vi "GetDataEventProperties.vi"(8 "error in (no error)":errorcluster, 9 "data":T2, 10 "Ir Data Event":T7, 11 "config":T6) -> (0 "error out":errorcluster, 1 "Timestamp":i64, 2 "Props":T1[](array[typedef]), 3 "AssetNodeId":string)   [LabVIEW 2017, in "IrDataEventCreator.lvlib"]
uses:
  <vilib>/addons/InsightCM/Devices/Shared/Ir/IrDataEventCreator/IrDataEventCreator.lvlib
  <vilib>/addons/InsightCM/Devices/Shared/Ir/IrDataEventCreator/controls/IrDataEvent.ctl
  <vilib>/addons/InsightCM/Devices/Shared/Common/DataEvent/controls/EventReference.ctl
  <vilib>/addons/InsightCM/Devices/Shared/Common/DataEvent/controls/Event.ctl
  <vilib>/addons/InsightCM/MessageBus/Base/controls/DataEvent.ctl
  <vilib>/addons/InsightCM/MessageBus/Base/controls/KeyValuePair.ctl
  <vilib>/addons/InsightCM/Devices/Shared/Common/DataEvent/controls/DataSet.ctl
  <vilib>/addons/InsightCM/MessageBus/Base/controls/DataSetMetadata.ctl
  <vilib>/addons/InsightCM/MessageBus/Base/controls/TrendPoint.ctl
  <vilib>/addons/InsightCM/MessageBus/Base/controls/TrendAlarmUpdate.ctl
  <vilib>/addons/InsightCM/MessageBus/Base/controls/TrendAlarmTransition.ctl
  <vilib>/addons/PointValueMap/controls/PointMap.ctl
  <vilib>/addons/InsightCM/Devices/Shared/Ir/IrDataEventCreator/controls/config.ctl
  <vilib>/addons/InsightCM/Devices/Shared/Common/DataFlow/controls/Data.ctl
  <vilib>/addons/InsightCM/Utilities/DataAccessors/controls/wfmSGL_DVR.ctl
  <vilib>/addons/InsightCM/Devices/Shared/Common/DataFlow/controls/Type.ctl
  <vilib>/addons/InsightCM/Utilities/PropertyHelpers/PropertyHelpers.lvlib
  <vilib>/addons/InsightCM/Devices/Shared/Common/DataEvent/DataEvent.lvlib
  <vilib>/addons/PointValueMap/PointValueMap.lvlib
  <vilib>/addons/InsightCM/Devices/Shared/Common/DataFlow/DataFlow.lvlib
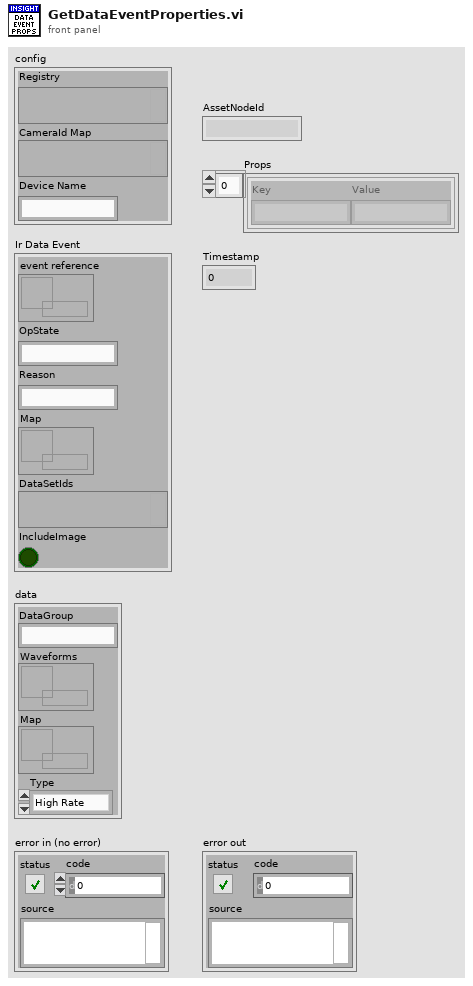
[diagram p1: front panel]
types:
  T1 = typedef "KeyValuePair.ctl" = cluster{"Key":string, "Value":string}
  T2 = typedef "DataFlow.lvlib/Data.ctl" = cluster{"DataGroup":string, "Waveforms":T3, "Map":T4, "Type":T5}
  T3 = typedef "wfmSGL_DVR.ctl" = refnum<data-value>
  T4 = typedef "PointValueMap.lvlib/PointMap.ctl" = refnum<data-value>
  T5 = typedef "DataFlow.lvlib/Type.ctl" = enum16{"High Rate", "Low Rate", "Burst Mode"}
  T6 = typedef "IrDataEventCreator.lvlib/config.ctl" = cluster{"Registry":variant, "CameraId Map":variant, "Device Name":string}
  T7 = typedef "IrDataEventCreator.lvlib/IrDataEvent.ctl" = cluster{"event reference":T8, "OpState":string, "Reason":string, "Map":T4, "DataSetIds":variant, "IncludeImage":bool}
  T8 = typedef "DataEvent.lvlib/EventReference.ctl" = refnum<data-value>
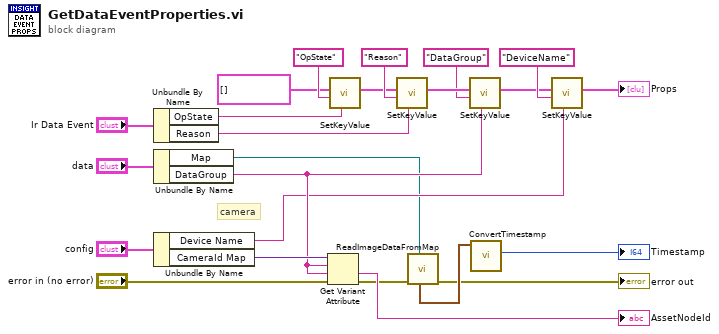
[diagram p0: block diagram]
diagram:
  # "camera"
  n1 = Unbundle By Name("Ir Data Event") -> ("OpState"=w6:string, "Reason"=w16:string)
  n2 = Unbundle By Name("data") -> ("Map"=w4:T4, "DataGroup"=w13:string)
  n3 = Unbundle By Name("config") -> ("Device Name"=w11:string, "CameraId Map"=w22:variant)
  n4 = Get Variant Attribute(Variant=w22, name=w13, default value (empty Variant)=w13, error in="error in (no error)") -> (value=→"AssetNodeId":string, error out=w2:errorcluster)  [unwired: 2 out]
  n5 = call <vilib>:"SetKeyValue.vi"("value"=w6, "key"="OpState", "key value pairs"=T1[] []) -> ("key value pairs out"=w8:T1[])  [unwired: 8 in]
  n6 = call <vilib>:"SetKeyValue.vi"("value"=w16, "key"="Reason", "key value pairs"=w8) -> ("key value pairs out"=w15:T1[])  [unwired: 8 in]
  n7 = call <vilib>:"ReadImageDataFromMap.vi"("map"=w4, "error in (no error)"=w2) -> ("error out"=→"error out":errorcluster, "image timestamp"=w3:timestamp)  [unwired: 3 in, 5 out]
  n8 = call <vilib>:"SetKeyValue.vi"("value"=w13, "key"="DataGroup", "key value pairs"=w15) -> ("key value pairs out"=w10:T1[])  [unwired: 8 in]
  n9 = call <vilib>:"ConvertTimestamp.vi"("Time Stamp"=w3) -> ("Timestamp out"=→"Timestamp":i64)  [unwired: 10 in]
  n10 = call <vilib>:"SetKeyValue.vi"("value"=w11, "key"="DeviceName", "key value pairs"=w10) -> ("key value pairs out"=→"Props":T1[])  [unwired: 8 in]
